vi "Temperature Min Read Array.vi"(8 "error in":errorcluster, 11 "Climate Chamber in":refnum<class "Climate Chamber.lvclass">) -> (0 "error out":errorcluster, 1 "Changed or First Call?":bool, 2 "Temperature Min SP":dbl[](array[numeric]), 3 "Climate Chamber out":refnum<class "Climate Chamber.lvclass">)   [LabVIEW 2023, in "Climate Chamber.lvclass"]
uses:
  Climate Chamber.lvclass
  Climate Chamber.lvclass/Climate Chamber.ctl
  Low Level Capabilities/Temperature/Temperature Limit/Temperature Limit.lvclass
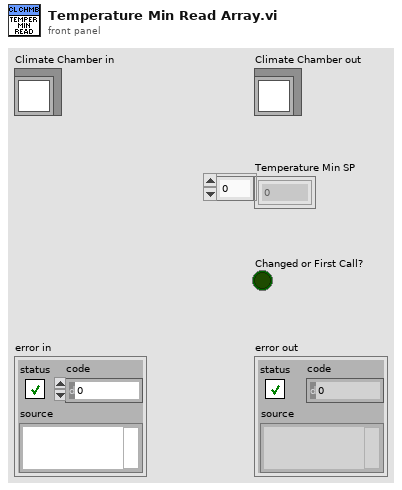
[diagram p1: front panel]
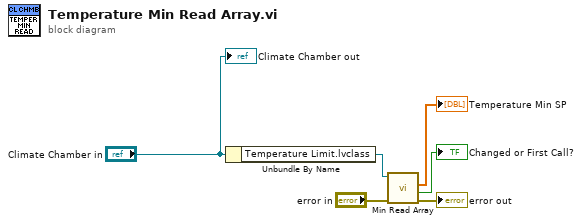
[diagram p0: block diagram]
diagram:
  n1 = Unbundle By Name("Climate Chamber in") -> ("Temperature Limit.lvclass"=w5:refnum<class "Temperature Limit.lvclass">)
  n2 = call-dynamic "Min Read Array.vi"("error in"="error in", "Min Temperature Limit in"=w5) -> ("error out"=→"error out":errorcluster, "Changed or First Call?"=→"Changed or First Call?":bool, "Temperature Min SP"=→"Temperature Min SP":dbl[])  [unwired: 6 in, 1 out]
  "Climate Chamber out" <- "Climate Chamber in"
